vi "Test Flatten to string setup for RFP.vi"() -> ()   [LabVIEW 2022 SP3]
uses:
  Anemometry/Anemometry Sub Vis/Data_plotting_vis/All_Setup.ctl
panel:
  in  "Save?":bool
  in  "Setup filename":string="hello1"
  in  "Filename Out":path=path "Z:/2019/Paul_Hayden_Desk/Paul_Hayden/Preferences/Results_File_Plotter_Setups/PAUL-HAYDEN-PC_Current_Setup.xls"
  out "value":T1={"Result files to read"=[], "Template"=path "", "Transpose"=FALSE, "Additional X Values"=[], "Additional Y Values"=[], "Output Filename"=path "", "Create Picture Vi Name"="Intensity plot jpg.vi", "Intensity Plot?"=FALSE, "Multi Ordinate"=[], "Abscissa String"="Intensity plot jpg.vi", "Filter Array"=[], "Filter Bins 1 Strings"=[""], "Filter Bins 2 Strings"=[""], "Filters 3 onwards"=[], "nRows"=0} {"Additional Y Values" format="%.2f"; "Additional X Values" format="%.2f"}
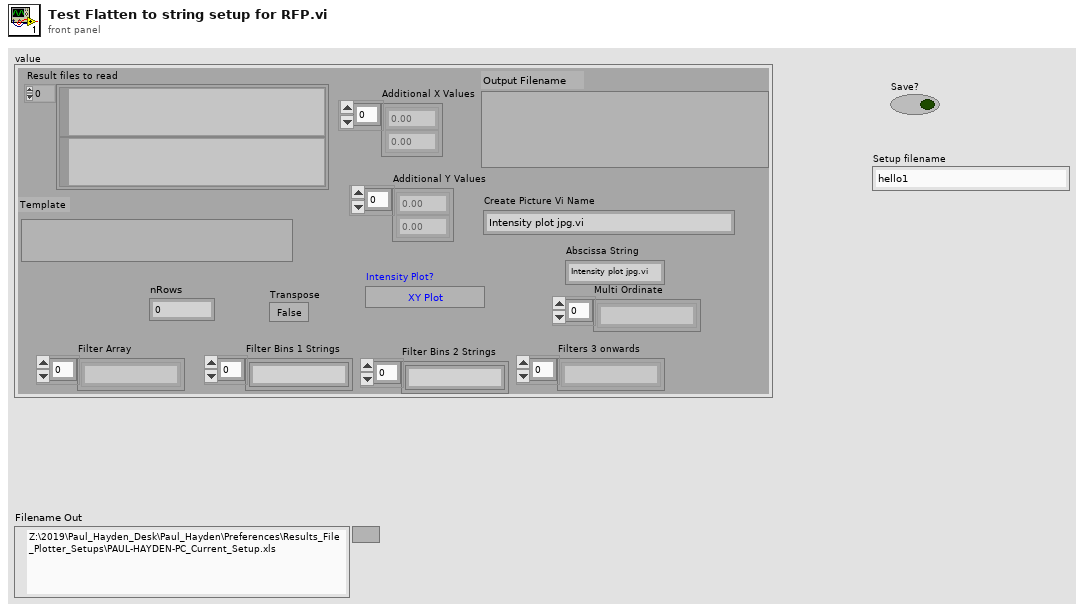
[diagram p1: front panel]
types:
  T1 = typedef "All_Setup.ctl" = cluster{"Result files to read":path[], "Template":path, "Transpose":bool, "Additional X Values":dbl[], "Additional Y Values":dbl[], "Output Filename":path, "Create Picture Vi Name":string, "Intensity Plot?":bool, "Multi Ordinate":string[], "Abscissa String":string, "Filter Array":string[], "Filter Bins 1 Strings":string[], "Filter Bins 2 Strings":string[], "Filters 3 onwards":string[], "nRows":i32}
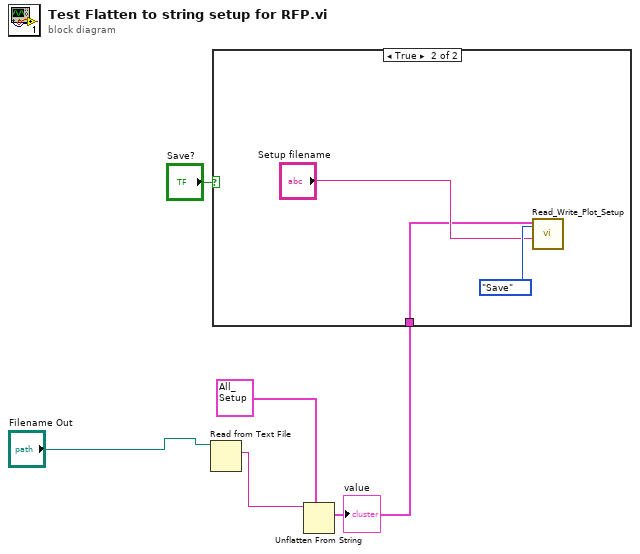
[diagram p0: block diagram]
diagram:
  n1 = Read from Text File(file (use dialog)="Filename Out") -> (text=w5:string)  [unwired: 3 in, 3 out]
  n2 = Unflatten From String(type=T1 {"Result files to read"=[], "Template"=path "", "Transpose"=FALSE, "Additional X Values"=[], "Additional Y Values"=[], "Output Filename"=path "", "Create Picture Vi Name"="Intensity plot jpg.vi", "Intensity Plot?"=FALSE, "Multi Ordinate"=[], "Abscissa String"="Intensity plot jpg.vi", "Filter Array"=["", "", "", "", "", ""], "Filter Bins 1 Strings"=[""], "Filter Bins 2 Strings"=[""], "Filters 3 onwards"=[], "nRows"=0} ("Cluster"), binary string=w5) -> (value=w2:T1)  [unwired: 1 in, 4 out]
  "value" <- w2
  n3 = case shown="True" "Save?" {
    tunnel: w2 -> [_ w6]
    frame False {
    }
    frame True {
      n4 = call "Read_Write_Plot_Setup.vi"("Mode"=enum16{"Load", "Save"}."Save", "Setup filename"="Setup filename", "Cluster"=w6) -> ()  [unwired: 6 in, 3 out]
    }
  }
